vi "Get Column Headers.vi"(8 "error in (no error)":errorcluster, 11 "Multicolumn List Box View Model In":refnum<class "Multicolumn List Box View Model.lvclass">) -> (0 "error out":errorcluster, 2 "Header Strings":string[](array[string]), 3 "Multicolumn List Box View Model Out":refnum<class "Multicolumn List Box View Model.lvclass">)   [LabVIEW 2020, in "Multicolumn List Box View Model.lvclass"]
uses:
  Multicolumn List Box View Model.lvclass
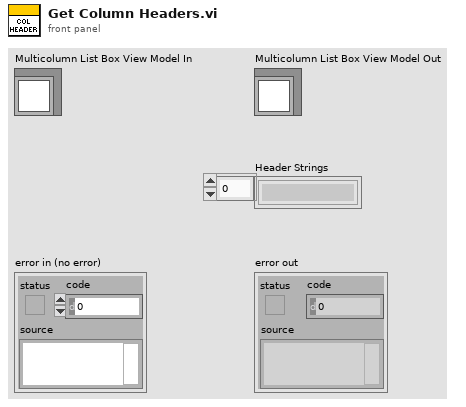
[diagram p1: front panel]
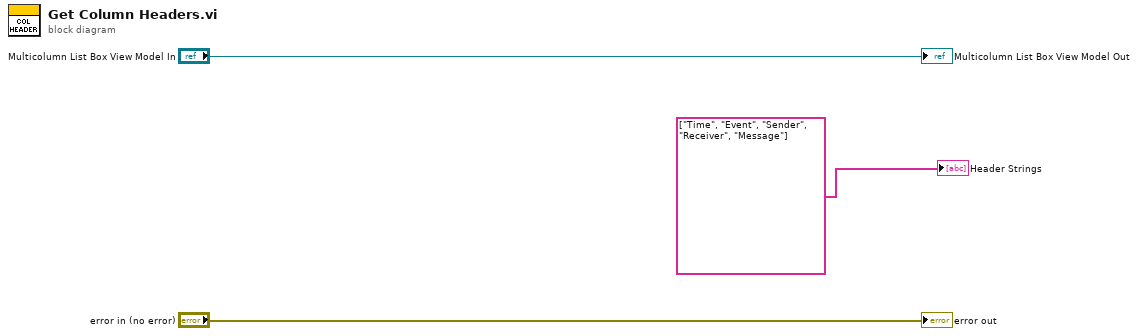
[diagram p0: block diagram]
diagram:
  "error out" <- "error in (no error)"
  "Multicolumn List Box View Model Out" <- "Multicolumn List Box View Model In"
  "Header Strings" <- string[] ["Time", "Event", "Sender", "Receiver", "Message"] ("Array")
